vi "ssh2_exec.vi"() -> ()   [LabVIEW 2013]
uses:
  <vilib>/Utility/sysdir.llb/System Directory Type.ctl
  libssh2.lvlib
panel:
  out "exitsignal":string
  out "Output":string
  out "exit status":i32
  in  "command":string="ping localhost -c 1"
  in  "password":string
  in  "username":string
  out "error out":errorcluster
  in  "hostname":string="localhost"
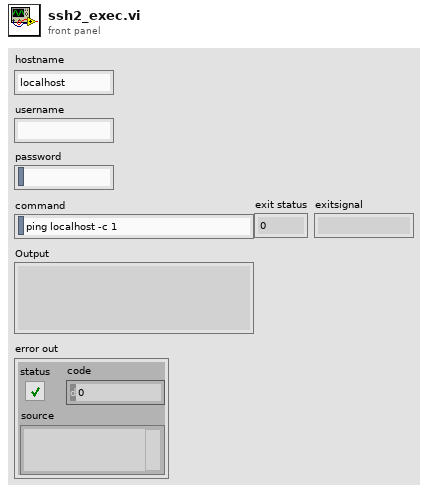
[diagram p1: front panel]
types:
  T1 = typedef "System Directory Type.ctl" = i32
  T2 = typedef "libssh2.lvlib/Session Refnum.ctl" = refnum<k1>
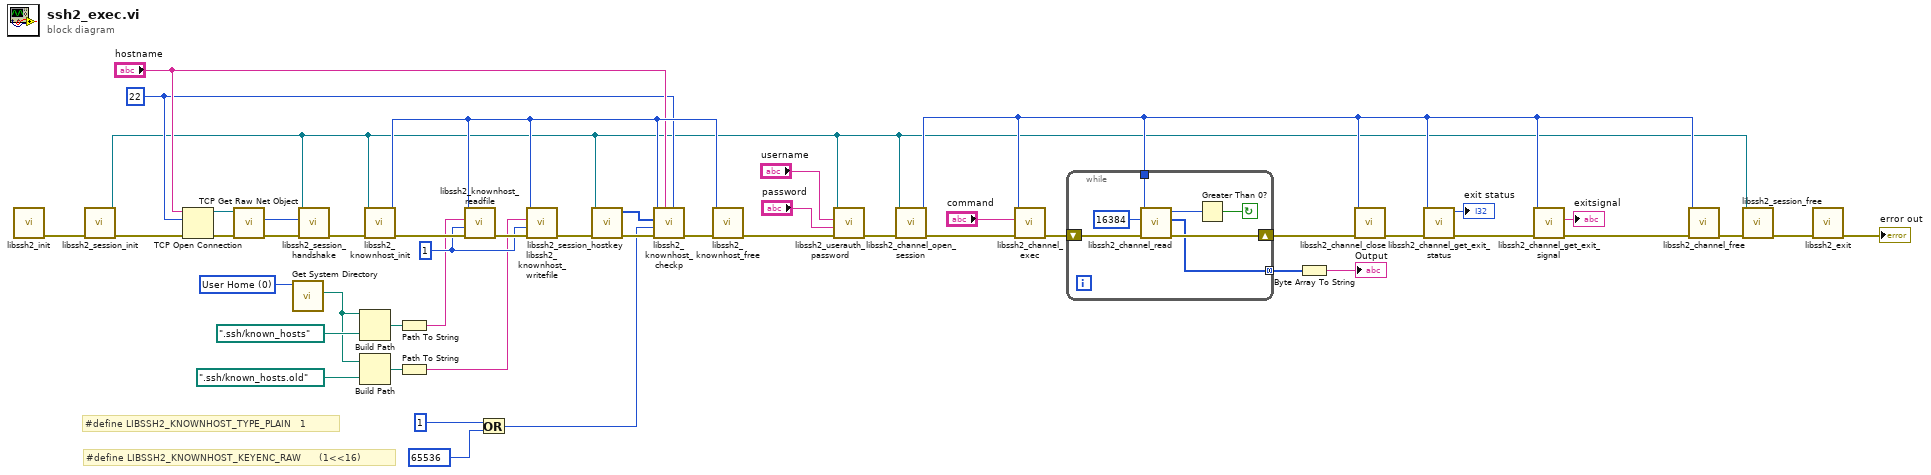
[diagram p0: block diagram]
diagram:
  w40 = T1 0 items=["User Home"=0, "User Desktop"=1, "User Documents"=2, "User Application Data"=3, "User Preferences"=4, "User Temporary"=5, "Public Documents"=6, "Public Application Data"=7, "Public Preferences"=8, "Public Cache"=13, "System Core Libraries"=9, "System Installed Libraries"=10, "Application Files"=11, "Boot Volume Root"=12] ("system directory type")
  w43 = 1 ("type")
  w19 = u16 22 ("remote port or service name")
  # "#define LIBSSH2_KNOWNHOST_KEYENC_RAW      (1<<16)"
  # "#define LIBSSH2_KNOWNHOST_TYPE_PLAIN   1"
  n1 = call "libssh2_init.vi"() -> ("error out"=w48:errorcluster)  [unwired: 10 in, 1 out]
  n2 = call "libssh2_session_init.vi"("error in (no error)"=w48) -> ("error out"=w47:errorcluster, "Session"=w1:T2)  [unwired: 9 in]
  n3 = TCP Open Connection(address="hostname", remote port or service name=w19, error in (no error)=w47) -> (connection ID=w29:refnum<k5>, error out=w30:errorcluster)  [unwired: 2 in]
  n4 = call <vilib>:"TCP Get Raw Net Object.vi"("error in (no error)"=w30, "connection ID"=w29) -> ("error out"=w28:errorcluster, "raw net object"=w27:u64)  [unwired: 7 in, 1 out]
  n5 = call <vilib>:"Get System Directory.vi"("system directory type"=w40) -> ("system directory"=w34:path)  [unwired: 10 in]
  n6 = call "libssh2_session_handshake.vi"("error in (no error)"=w28, "socket"=w27, "Session"=w1) -> ("error out"=w46:errorcluster)  [unwired: 7 in, 1 out]
  n7 = Build Path(base path=w34, name or relative path=path ".ssh/known_hosts") -> (appended path=w38:path)
  n8 = Build Path(base path=w34, name or relative path=path ".ssh/known_hosts.old") -> (appended path=w35:path)
  n9 = call "libssh2_knownhost_init.vi"("error in (no error)"=w46, "Session"=w1) -> ("error out"=w45:errorcluster, "return value"=w23:u64)  [unwired: 8 in]
  n10 = Path To String(path=w38) -> (string=w37:string)
  n11 = Path To String(path=w35) -> (string=w33:string)
  n12 = call "libssh2_knownhost_readfile.vi"("error in (no error)"=w45, "type"=w43, "filename"=w37, "hosts"=w23) -> ("error out"=w44:errorcluster)  [unwired: 6 in, 1 out]
  n13 = Or(x=1, y=65536) -> (x .or. y?=w21:i32)
  n14 = call "libssh2_knownhost_writefile.vi"("error in (no error)"=w44, "type"=w43, "filename"=w33, "hosts"=w23) -> ("error out"=w26:errorcluster)  [unwired: 6 in, 1 out]
  n15 = call "libssh2_session_hostkey.vi"("error in (no error)"=w26, "Session"=w1) -> ("error out"=w25:errorcluster, "return value"=w22:u8[])  [unwired: 7 in, 1 out]
  n16 = call "libssh2_knownhost_checkp.vi"("port"=w19, "host"="hostname", "error in (no error)"=w25, "typemask"=w21, "key"=w22, "hosts"=w23) -> ("error out"=w24:errorcluster)  [unwired: 2 in, 3 out]
  n17 = call "libssh2_knownhost_free.vi"("error in (no error)"=w24, "hosts"=w23) -> ("error out"=w18:errorcluster)  [unwired: 9 in]
  n18 = call "libssh2_userauth_password.vi"("error in (no error)"=w18, "password"="password", "username"="username", "Session"=w1) -> ("error out"=w17:errorcluster)  [unwired: 6 in, 1 out]
  n19 = call "libssh2_channel_open_session.vi"("error in (no error)"=w17, "Session"=w1) -> ("error out"=w14:errorcluster, "return value"=w5:u64)  [unwired: 8 in]
  n20 = call "libssh2_channel_exec.vi"("error in (no error)"=w14, "command"="command", "channel"=w5) -> ("error out"=w13:errorcluster)  [unwired: 7 in, 1 out]
  n21 = while {
    tunnel: w5 -> [w52]
    tunnel: [w49] -> w3 mode=concatenating
    shift-right: [w54] -> w11
    shift-left: w13 -> [w55]
    stop <- w50 continue-if-true
    n22 = call "libssh2_channel_read.vi"("error in (no error)"=w55, "buflen"=u64 16384, "channel"=w52) -> ("error out"=w54:errorcluster, "buf"=w49:u8[], "return value"=w51:i64)  [unwired: 6 in]
    n23 = Greater Than 0?(x=w51) -> (x > 0?=w50:bool)
  }
  n24 = Byte Array To String(unsigned byte array=w3) -> (string=→"Output":string)
  n25 = call "libssh2_channel_close.vi"("error in (no error)"=w11, "channel"=w5) -> ("error out"=w10:errorcluster)  [unwired: 8 in, 1 out]
  n26 = call "libssh2_channel_get_exit_status.vi"("error in (no error)"=w10, "channel"=w5) -> ("error out"=w8:errorcluster, "return value"=→"exit status":i32)  [unwired: 8 in]
  n27 = call "libssh2_channel_get_exit_signal.vi"("error in (no error)"=w8, "channel"=w5) -> ("error out"=w7:errorcluster, "exitsignal"=→"exitsignal":string)  [unwired: 5 in, 3 out]
  n28 = call "libssh2_channel_free.vi"("error in (no error)"=w7, "channel"=w5) -> ("error out"=w6:errorcluster)  [unwired: 8 in, 1 out]
  n29 = call "libssh2_session_free.vi"("error in (no error)"=w6, "Session"=w1) -> ("error out"=w42:errorcluster)  [unwired: 8 in, 1 out]
  n30 = call "libssh2_exit.vi"("error in (no error)"=w42) -> ("error out"=→"error out":errorcluster)  [unwired: 10 in]
